vi "Facade.vi"(0 "Data In":T4=variant(dbl 0.0), 2 "Display State In":T2, 3 "Container State":T3) -> (6 "Data Out":T4=variant(dbl 0.0), 7 "Display State Out":T2, 8 "Action":T1)   [LabVIEW 2017, in "Variant Tree API.lvlib" / "Variant Tree.xctl"]
uses:
  Variant Tree.xctl
  Data.ctl
  <vilib>/_xctls/Container State.ctl
  State.ctl
  <vilib>/_xctls/Action.ctl
  <vilib>/National Instruments/Variant Data Manipulation/Path API/Write Value at Path(String).vi
  <vilib>/_xctls/XControlSupport.lvlib
  Variant Tree API.lvlib
  <vilib>/National Instruments/Variant JSON API/Variant JSON API.lvlib
  <vilib>/Utility/Data Type/NI_Data Type.lvlib
  <vilib>/National Instruments/Variant Data Manipulation/Variant Data Manipulation.lvlib
panel:
  in  "Tree":string(tree)
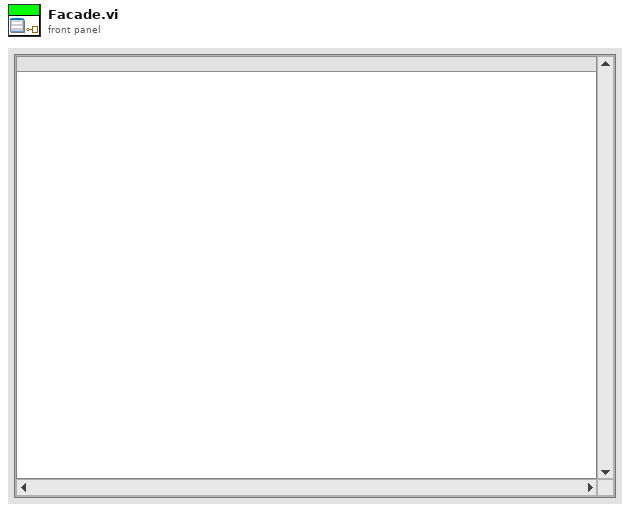
[diagram p1: front panel]
types:
  T1 = typedef "XControlSupport.lvlib/Action.ctl" = cluster{"Data Changed?":bool, "State Changed?":bool, "Action Name":string}
  T2 = typedef "Variant Tree API.lvlib/Variant Tree.xctl/State.ctl" = cluster{"Numeric":dbl}
  T3 = typedef "XControlSupport.lvlib/Container State.ctl" = cluster{"Indicator?":bool, "Run Mode?":bool, " Refnum":refnum<vi>}
  T4 = typedef "Variant Tree API.lvlib/Variant Tree.xctl/Data.ctl" = variant
  T5 = typedef "NI_Data Type.lvlib/Data Type.ctl" = enum8{"Invalid Type", "Void", "I8", "I16", "I32", "I64", "U8", "U16", "U32", "U64", "Single Float", "Double Float", "Extended Float", "Single Complex", "Double Complex", "Extended Complex", "Enum U8", "Enum U16", "Enum U32", "Enum U64", "Single Float With Unit", "Double Float With Unit", "Extended Float With Unit", "Single Complex with Unit", "Double Complex with Unit", "Extended Complex with Unit", "Boolean", "String", "Path", "Picture", "Tag", "Array", "Cluster", "Variant", "LV Variant", "Waveform", "Timestamp", "Digital Waveform", "Digital Data", "ExpressData", "Refnum", "External Data", "VI", "Poly VI", "LabVIEW Class Instance", "Fixed Point"}
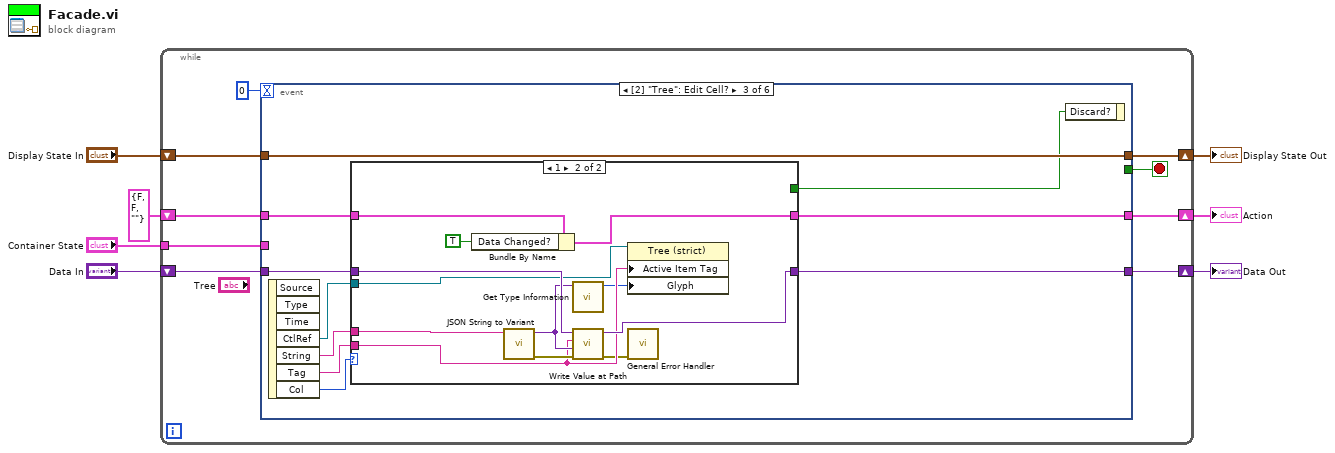
[diagram p0: block diagram]
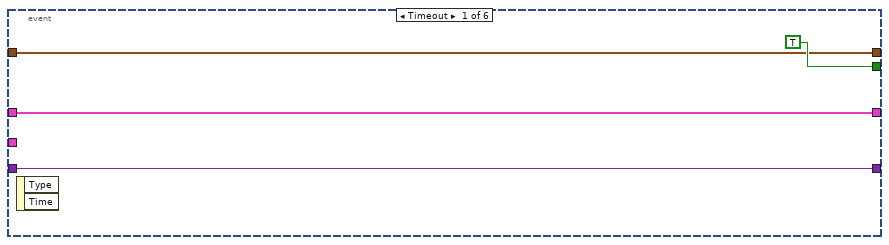
[diagram p2: hidden frame]
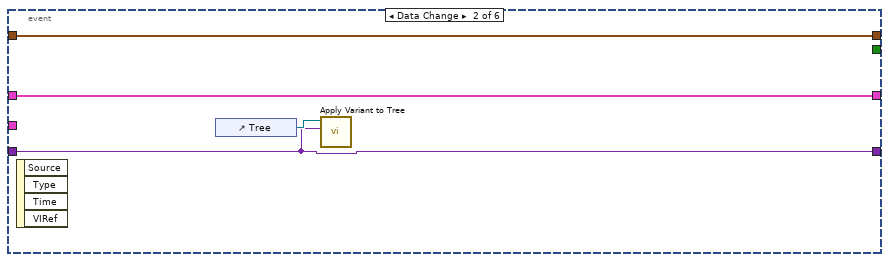
[diagram p3: hidden frame]
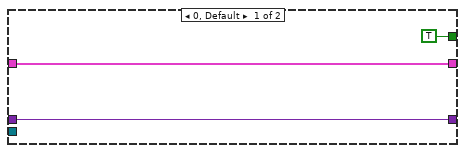
[diagram p4: hidden frame]
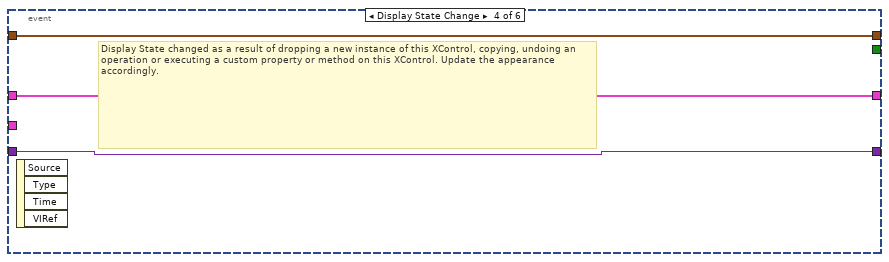
[diagram p5: hidden frame]
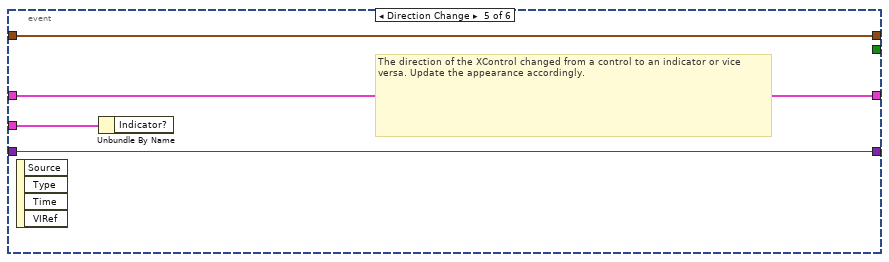
[diagram p6: hidden frame]
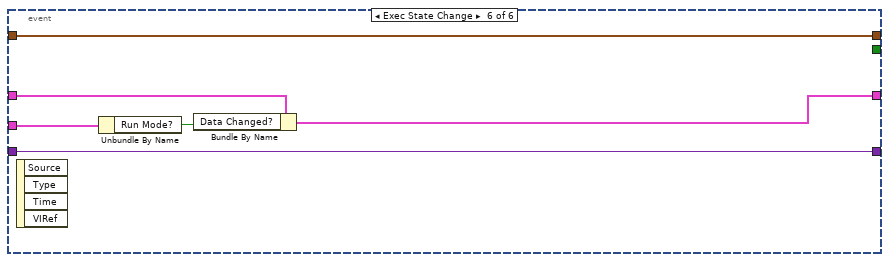
[diagram p7: hidden frame]
diagram:
  n1 = while {
    shift-right: [w15] -> w4
    shift-left: "Display State In" -> [w16]
    tunnel: "Container State" -> [w12]
    shift-right: [w10] -> w7
    shift-left: "Data In" -> [w11]
    shift-right: [w8] -> w2
    shift-left: T1 {"Data Changed?"=FALSE, "State Changed?"=FALSE, "Action Name"=""} ("Action") -> [w9]
    stop <- w14 stop-if-true
    n2 = event shown="[2] \"Tree\": Edit Cell?" {
      selector: _ -> [_ _ _ _ _ _]
      dyn-events: _ -> [_ _ _ _ _ _]
      timeout: 0 -> [_ _ _ _ _ _]
      tunnel: w16 -> [w19 w24 w34 w52 w55 w61]
      tunnel: [w19 w24 w34 w52 w55 w61] -> w15
      tunnel: [TRUE _ _ _ _ _] -> w14
      tunnel: w12 -> [_ _ _ _ w56 w62]
      tunnel: w11 -> [w18 w22 w30 w51 w54 w60]
      tunnel: [w18 w22 w29 w51 w54 w60] -> w10
      tunnel: w9 -> [w17 w21 w26 w50 w53 w58]
      tunnel: [w17 w21 w25 w50 w53 w57] -> w8
      event Timeout {
        n3 = event-data() -> ()  [unwired: 1 in, 2 out]
      }
      event Data Change {
        n4 = event-data() -> ()  [unwired: 1 in, 4 out]
        n5 = control-ref of="Tree"() -> (w23:refnum<vi>)
        n6 = call "Apply Variant to Tree.vi"("Variant"=w22, "TreeControl in"=w23) -> ()  [unwired: 8 in, 2 out]
      }
      event "Tree": Edit Cell? {
        n7 = event-data() -> ("CtlRef"=w27:refnum<vi>, "String"=w28:string, "Tag"=w31:string, "Col"=w33:i32)  [unwired: 1 in, 3 out]
        n8 = case shown="1" w33 {
          tunnel: [TRUE _] -> w32
          tunnel: w31 -> [_ w43]
          tunnel: w30 -> [w36 w49]
          tunnel: [w36 w47] -> w29
          tunnel: w28 -> [_ w48]
          tunnel: w27 -> [_ w44]
          tunnel: w26 -> [w35 w40]
          tunnel: [w35 w39] -> w25
          frame 0, Default {
          }
          frame 1 {
            n9 = Bundle By Name(cluster=w40, "Data Changed?"=TRUE) -> (w39:T1)
            n10 = call <vilib>:"JSON String to Variant.vi"("JSON String"=w48) -> ("error out"=w46:errorcluster, "Variant out"=w45:variant)  [unwired: 9 in]
            n11 = call <vilib>:"Get Type Information.vi"("Variant"=w45) -> ("Type"=w42:T5)  [unwired: 6 in, 4 out]
            n12 = call-poly <vilib>:"Write Value at Path.vi"("error in (no error)"=w46, "Element in"=w45, "Path String"=w43, "Variant in"=w49) -> ("error out"=w41:errorcluster, "Variant out"=w47:variant)  [unwired: 6 in]
            n13 = property class="Tree (strict)"(reference=w44, "Active Item Tag"=w43, "Glyph"=w42) -> ()  [unwired: 1 in, 2 out]
            n14 = call <vilib>:"General Error Handler.vi"("error in (no error)"=w41) -> ()  [unwired: 10 in, 5 out]
          }
        }
        n15 = event-data("Discard?"=w32) -> ()  [unwired: 1 in, 1 out]
      }
      event Display State Change {
        # "Display State changed as a result of dropping a new instance of this XControl, copying, undoing an operation or executing a custom property or method on this XControl. Update the appearance accordingly."
        n16 = event-data() -> ()  [unwired: 1 in, 4 out]
      }
      event Direction Change {
        # "The direction of the XControl changed from a control to an indicator or vice versa. Update the appearance accordingly."
        n17 = event-data() -> ()  [unwired: 1 in, 4 out]
        n18 = Unbundle By Name(w56) -> ()  [unwired: 1 out]
      }
      event Exec State Change {
        n19 = event-data() -> ()  [unwired: 1 in, 4 out]
        n20 = Unbundle By Name(w62) -> ("Run Mode?"=w59:bool)
        n21 = Bundle By Name(cluster=w58, "Data Changed?"=w59) -> (w57:T1)
      }
    }
  }
  "Display State Out" <- w4
  "Data Out" <- w7
  "Action" <- w2
